vi "stop.vi"(8 "error in (no error)":errorcluster, 11 "TrajectoryMG100122GenericFPGA in":refnum<class "TrajectoryMG100122GenericFPGA.lvclass">) -> (0 "error out":errorcluster, 3 "TrajectoryMG100122GenericFPGA out":refnum<class "TrajectoryMG100122GenericFPGA.lvclass">)   [LabVIEW 2010, in "TrajectoryMG100122GenericFPGA.lvclass"]
uses:
  TrajectoryMG100122GenericFPGA.lvclass
  FPGAWrapper/GenericFPGAWrapper/GenericFPGAWrapper/GenericFPGAWrapper.lvclass
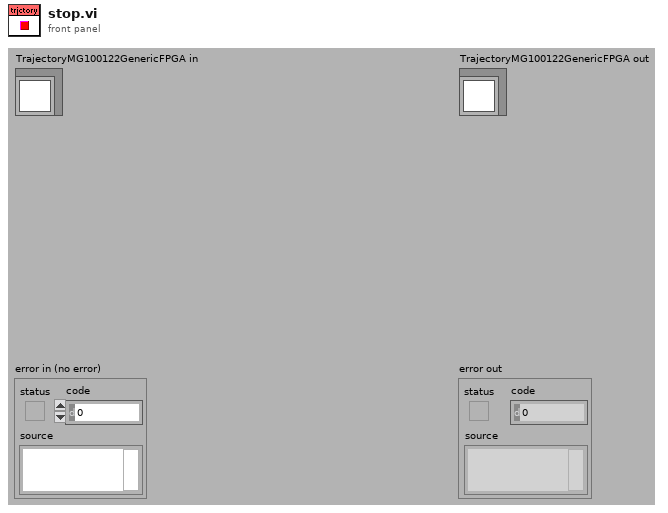
[diagram p1: front panel]
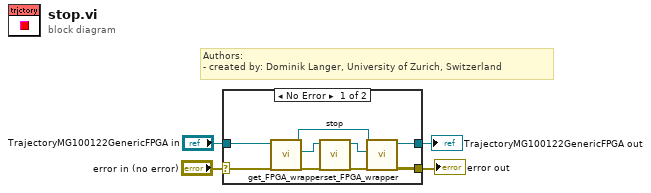
[diagram p0: block diagram]
diagram:
  # "Authors: \n- created by: Dominik Langer, University of Zurich, Switzerland"
  n1 = case shown="No Error" "error in (no error)" {
    selector: "error in (no error)" -> [w12 w15]
    tunnel: [w8 w15] -> w3
    tunnel: [w5 w14] -> w4
    tunnel: "TrajectoryMG100122GenericFPGA in" -> [w13 w14]
    frame No Error {
      n2 = call-dynamic "get_FPGA_wrapper.vi"("error in (no error)"=w12, "TrajectoryMG100122GenericFPGA in"=w13) -> ("error out"=w11:errorcluster, "GenericFPGAWrapper.lvclass"=w10:refnum<class "GenericFPGAWrapper.lvclass">, "TrajectoryMG100122GenericFPGA out"=w6:refnum<class "TrajectoryMG100122GenericFPGA.lvclass">)  [unwired: 7 in]
      n3 = call-dynamic "stop.vi"("error in (no error)"=w11, "GenericFPGAWrapper in"=w10) -> ("error out"=w9:errorcluster, "GenericFPGAWrapper out"=w7:refnum<class "GenericFPGAWrapper.lvclass">)  [unwired: 8 in]
      n4 = call-dynamic "set_FPGA_wrapper.vi"("error in (no error)"=w9, "GenericFPGAWrapper.lvclass"=w7, "TrajectoryMG100122GenericFPGA in"=w6) -> ("error out"=w8:errorcluster, "TrajectoryMG100122GenericFPGA out"=w5:refnum<class "TrajectoryMG100122GenericFPGA.lvclass">)  [unwired: 7 in]
    }
    frame Error {
    }
  }
  "error out" <- w3
  "TrajectoryMG100122GenericFPGA out" <- w4
